vi "pattern_results.vi"(11 "Boolean":bool) -> (3 "String":string)   [LabVIEW 2013]
uses:
  <vilib>/Utility/miscctls.llb/LVBoundsTypeDef.ctl
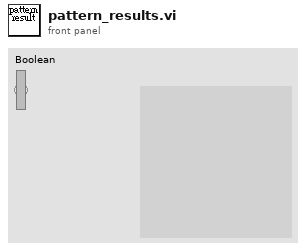
[diagram p1: front panel]
types:
  T1 = typedef "LVBoundsTypeDef.ctl" = cluster{"Width":u32, "Height":u32}
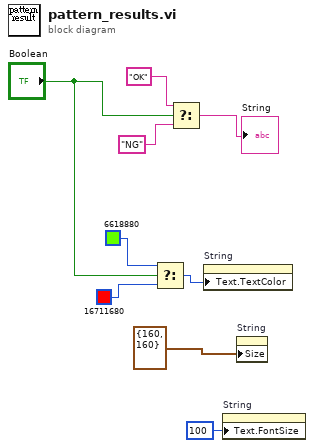
[diagram p0: block diagram]
diagram:
  n1 = Select(t=u32 6618880, s="Boolean", f=u32 16711680) -> (s? t:f=w2:u32)
  n2 = Select(t="OK", s="Boolean", f="NG") -> (s? t:f=→"String":string)
  n3 = property on="String" class="Str"("Text.TextColor"=w2) -> ()  [unwired: 2 in, 2 out]
  n4 = property on="String" class="Str"("Text.FontSize"=u32 100 ("Text.Font:Size")) -> ()  [unwired: 2 in, 2 out]
  n5 = property on="String" class="Str"("Size"=T1 {"Width"=160, "Height"=160}) -> ()  [unwired: 2 in, 2 out]
